vi "lv_icon_launcher.vi"(10 "Color icon in":T1, 11 "BW icon in":T1) -> (0 "Error code out":i32, 2 "Color icon out":T1, 3 "BW icon out":T1)   [LabVIEW 2020]
uses:
  <vilib>/picture/picture.llb/imagedata.ctl
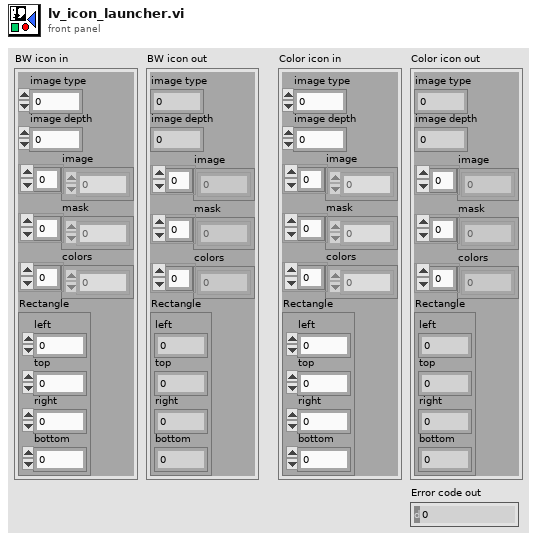
[diagram p1: front panel]
types:
  T1 = typedef "imagedata.ctl" = cluster{"image type":i32, "image depth":i32, "image":u8[], "mask":u8[], "colors":u32[], "Rectangle":cluster{"left":i16, "top":i16, "right":i16, "bottom":i16}}
  T2 = enum32{"Invalid", "Standard", "Closed", "Hidden", "Minimized", "Maximized"}
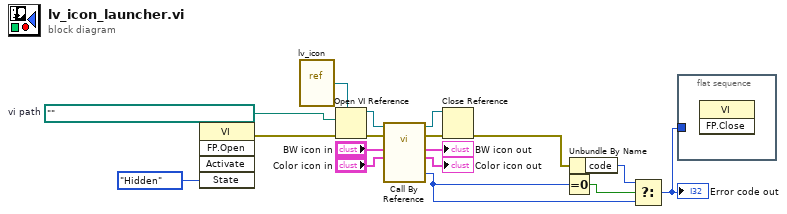
[diagram p0: block diagram]
diagram:
  w6 = path ""  # vi path
  n1 = invoke class="VI" method="FP.Open"("State"=T2."Hidden") -> (error out=w15:errorcluster)  [unwired: 4 in, 4 out]
  n2 = vi-ref "lv_icon.vi"() -> (w13:refnum<vi>)
  n3 = Open VI Reference(type specifier VI Refnum (for type only)=w13, vi path=w6, error in (no error)=w15) -> (vi reference=w12:refnum<vi>, error out=w17:errorcluster)  [unwired: 3 in]
  n4 = call-by-ref "Call By Reference"(reference=w12, error in=w17, "Color icon in"="Color icon in", "BW icon in"="BW icon in") -> (reference out=w11:refnum<vi>, error out=w16:errorcluster, "Error code out"=w3:i32, "Color icon out"=→"Color icon out":T1, "BW icon out"=→"BW icon out":T1)  [unwired: 7 in]
  n5 = Close Reference(reference=w11, error in (no error)=w16) -> (error out=w14:errorcluster)
  n6 = Equal To 0?(x=w3) -> (x = 0?=w4:bool)
  n7 = Unbundle By Name(w14) -> ("code"=w2:i32)
  n8 = Select(t=w2, s=w4, f=w3) -> (s? t:f=w1:i32)
  "Error code out" <- w1
  n9 = flat-sequence {
    tunnel: w1 -> [_]
    frame #0 {
      n10 = invoke class="VI" method="FP.Close"() -> ()  [unwired: 3 in, 3 out]
    }
  }
